vi "Temp_v2.vi"(8 "error in":errorcluster, 10 "Read Task":string="BONTS_TEMP_AC_Feedback", 11 "Write Task":string="BONTS_Temp_AC_Input") -> (0 "error out":errorcluster, 3 "Temp Fdbk":dbl[](array[numeric]) format="%.2p")   [LabVIEW 2021]
uses:
  <vilib>/DAQmx/write.llb/DAQmx Write (Analog DBL 1Chan 1Samp).vi
  <vilib>/DAQmx/read.llb/DAQmx Read (Analog 1D Wfm NChan NSamp).vi
  <vilib>/DAQmx/miscellaneous.llb/DAQmx Fill In Error Info.vi
  <vilib>/measure/madcrms.llb/Basic Averaged DC-RMS for N Chan.vi
  <vilib>/measure/NI_MAPro.lvlib
panel:
  out "Output Signal":waveform(dbl)[](graph)=[{"t0"=timestamp(0 s since 1904-01-01), "dt"=0.001, "Y"=[]}]
  # "All measurements are in Volts DC"
  # "Temp In"
  # "0"
  # "1"
  # "2"
  # "3"
  # "4"
  # "5"
  # "0"
  # "This test steps up the voltage in 1s increments.\nThe increases in voltage goes back and forth\nbetween inputs A and C"
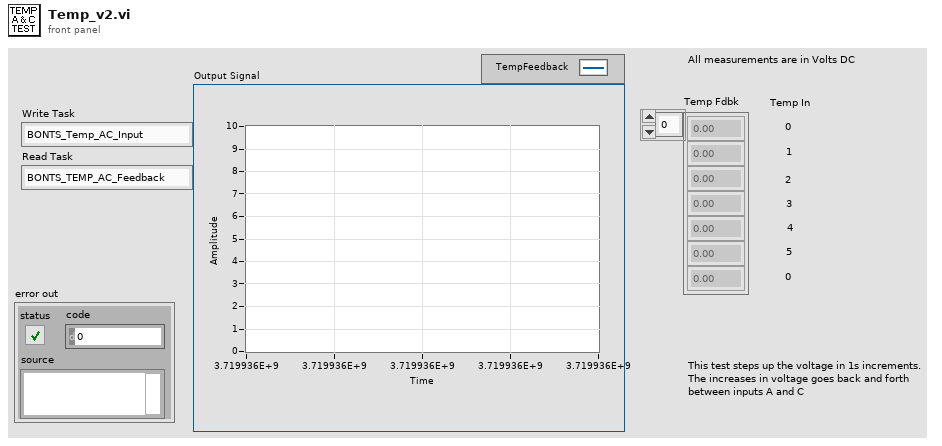
[diagram p1: front panel]
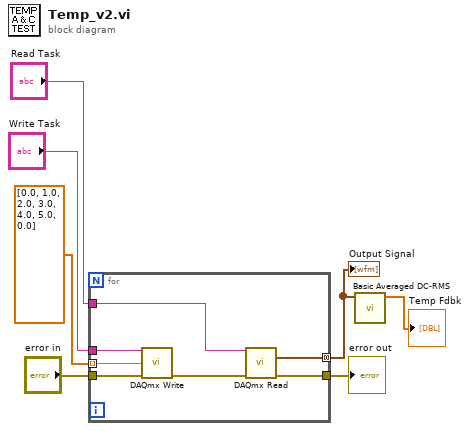
[diagram p0: block diagram]
diagram:
  n1 = for {
    tunnel: "Write Task" -> [w14]
    tunnel: "Read Task" -> [w13]
    tunnel: [w12] -> w1
    tunnel: dbl[] [0.0, 1.0, 2.0, 3.0, 4.0, 5.0, 0.0] -> [w11] mode=indexing
    tunnel: "error in" -> [w9]
    tunnel: [w8] -> w3 mode=concatenating
    n2 = call-poly <vilib>:"DAQmx Write.vi"("task/channels in"=w14, "data"=w11, "error in"=w9) -> ("error out"=w10:errorcluster)  [unwired: 10 in, 2 out]
    n3 = call-poly <vilib>:"DAQmx Read.vi"("task/channels in"=w13, "error in"=w10) -> ("data"=w8:waveform(dbl)[], "error out"=w12:errorcluster)  [unwired: 11 in, 1 out]
  }
  "Output Signal" <- w3
  "error out" <- w1
  n4 = call-poly <vilib>:"Basic Averaged DC-RMS.vi"("signals in"=w3) -> ("DC values"=→"Temp Fdbk":dbl[])  [unwired: 7 in, 3 out]
